vi "FindPropertyValue.vi"(10 "property":string, 11 "rows":string) -> (3 "value":string)   [LabVIEW 2016]
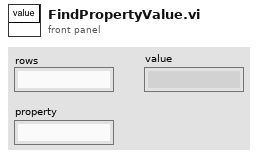
[diagram p1: front panel]
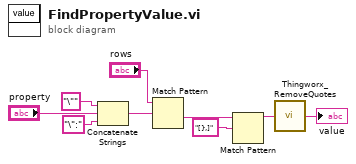
[diagram p0: block diagram]
diagram:
  n1 = Concatenate Strings("\"" ("string"), "property", "\":" ("string")) -> (w4:string)
  n2 = Match Pattern(string="rows", regular expression=w4) -> (after substring=w5:string)  [unwired: 1 in, 3 out]
  n3 = Match Pattern(string=w5, regular expression="[},]") -> (before substring=w7:string)  [unwired: 1 in, 3 out]
  n4 = call "Thingworx_RemoveQuotes.vi"("Incoming string in"=w7) -> ("Incoming string out"=→"value":string)
